vi "FileAppenderConfigFromDTO.vi"(8 "error in (no error)":errorcluster, 11 "FileAppenderConfigDTO":T7={"common"={"id"="", "threshold"="INFO", "filter"={"mode"="Mirror", "levelMin"="INFO", "levelMax"="INFO", "tagPrefix"=""}, "queueBound"=0, "dropPolicy"="DropOldest"}, "rootFolder"="", "maxFileSize"=0, "maxFileCount"=0, "baseName"="", "extension"="", "delimiter"="", "calendarFolderTree"=FALSE, "useUTC"=FALSE}) -> (0 "error out":errorcluster, 3 "FileAppenderConfig":T1={"common"={"id"="", "threshold"=enum."INFO", "filter"={"mode"=enum."Mirror", "levelMin"=enum."INFO", "levelMax"=enum."INFO", "tagPrefix"=""}, "queueBound"=0, "dropPolicy"=enum."DropOldest"}, "rootFolder"=path "", "maxFileSize"=0, "maxFileCount"=0, "baseName"="", "extension"="", "delimiter"="", "calendarFolderTree"=FALSE, "useUTC"=FALSE})   [LabVIEW 2026, in "Lumberjack.lvlib"]
uses:
  Lumberjack.lvlib
  TypeDefs/Severity.ctl
  TypeDefs/FilterMode.ctl
  TypeDefs/Filter.ctl
  TypeDefs/DropPolicy.ctl
  TypeDefs/AppenderConfig.ctl
  TypeDefs/FileAppenderConfig.ctl
  TypeDefs/ConfigDTO/FilterDTO.ctl
  TypeDefs/ConfigDTO/AppenderConfigDTO.ctl
  TypeDefs/ConfigDTO/FileAppenderConfigDTO.ctl
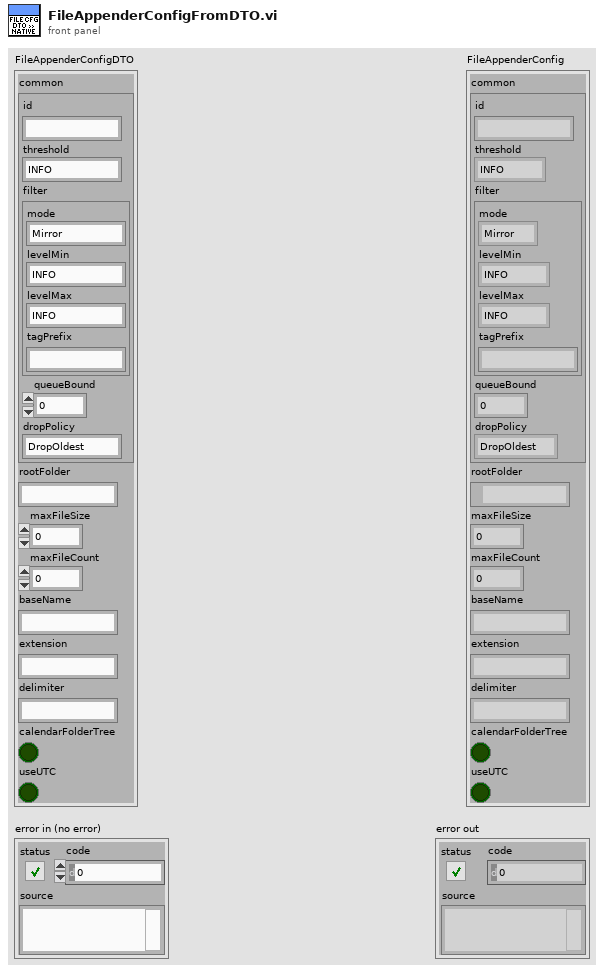
[diagram p1: front panel]
types:
  T1 = typedef "Lumberjack.lvlib/FileAppenderConfig.ctl" = cluster{"common":T2, "rootFolder":path, "maxFileSize":i64, "maxFileCount":i32, "baseName":string, "extension":string, "delimiter":string, "calendarFolderTree":bool, "useUTC":bool}
  T2 = typedef "Lumberjack.lvlib/AppenderConfig.ctl" = cluster{"id":string, "threshold":T3, "filter":T4, "queueBound":i32, "dropPolicy":T6}
  T3 = typedef "Lumberjack.lvlib/Severity.ctl" = enum16{"OFF", "FATAL", "ERROR", "WARN", "INFO", "DEBUG", "TRACE", "ALL"}
  T4 = typedef "Lumberjack.lvlib/Filter.ctl" = cluster{"mode":T5, "levelMin":T3, "levelMax":T3, "tagPrefix":string}
  T5 = typedef "Lumberjack.lvlib/FilterMode.ctl" = enum16{"Mirror", "Routed"}
  T6 = typedef "Lumberjack.lvlib/DropPolicy.ctl" = enum16{"DropOldest", "DropNewest", "LevelAware"}
  T7 = typedef "Lumberjack.lvlib/FileAppenderConfigDTO.ctl" = cluster{"common":T8, "rootFolder":string, "maxFileSize":i64, "maxFileCount":i32, "baseName":string, "extension":string, "delimiter":string, "calendarFolderTree":bool, "useUTC":bool}
  T8 = typedef "Lumberjack.lvlib/AppenderConfigDTO.ctl" = cluster{"id":string, "threshold":string, "filter":T9, "queueBound":i32, "dropPolicy":string}
  T9 = typedef "Lumberjack.lvlib/FilterDTO.ctl" = cluster{"mode":string, "levelMin":string, "levelMax":string, "tagPrefix":string}
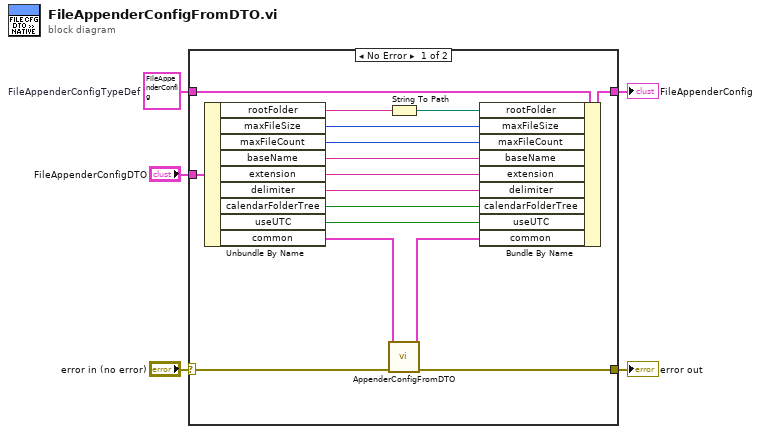
[diagram p0: block diagram]
diagram:
  w5 = T1 {"common"={"id"="", "threshold"=enum."INFO", "filter"={"mode"=enum."Mirror", "levelMin"=enum."INFO", "levelMax"=enum."INFO", "tagPrefix"=""}, "queueBound"=0, "dropPolicy"=enum."DropOldest"}, "rootFolder"=path "", "maxFileSize"=0, "maxFileCount"=0, "baseName"="", "extension"="", "delimiter"="", "calendarFolderTree"=FALSE, "useUTC"=FALSE}  # FileAppenderConfigTypeDef
  n1 = case shown="No Error" "error in (no error)" {
    selector: "error in (no error)" -> [w21 w23]
    tunnel: [w18 w23] -> w1
    tunnel: "FileAppenderConfigDTO" -> [w19 _]
    tunnel: [w20 w22] -> w2
    tunnel: w5 -> [w17 w22]
    frame No Error {
      n2 = Unbundle By Name(w19) -> ("rootFolder"=w7:string, "maxFileSize"=w16:i64, "maxFileCount"=w15:i32, "baseName"=w14:string, "extension"=w13:string, "delimiter"=w12:string, "calendarFolderTree"=w11:bool, "useUTC"=w10:bool, "common"=w9:T8)
      n3 = String To Path(string=w7) -> (path=w6:path)
      n4 = call "AppenderConfigFromDTO.vi"("error in (no error)"=w21, "AppenderConfigDTO"=w9) -> ("error out"=w18:errorcluster, "AppenderConfig"=w8:T2)  [unwired: 8 in]
      n5 = Bundle By Name(cluster=w17, "rootFolder"=w6, "maxFileSize"=w16, "maxFileCount"=w15, "baseName"=w14, "extension"=w13, "delimiter"=w12, "calendarFolderTree"=w11, "useUTC"=w10, "common"=w8) -> (w20:T1)
    }
    frame Error {
    }
  }
  "error out" <- w1
  "FileAppenderConfig" <- w2
